vi "add pre post build to project.vi"(8 "error in (no error)":errorcluster, 11 "Builder":refnum<class "Builder.lvclass">) -> (0 "error out":errorcluster, 3 "Builder out":refnum<class "Builder.lvclass">)   [LabVIEW 2024, in "Builder.lvclass"]
doc: "If the path is valid, adds the pre and post build spec action vis to the open lv project"
uses:
  builders/parent/Builder.lvclass
  builders/parent/Builder.lvclass/Builder.ctl
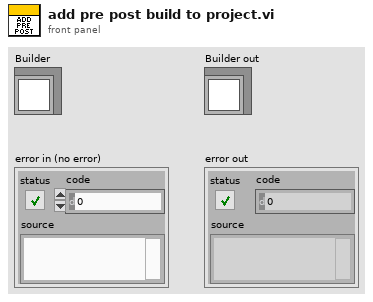
[diagram p1: front panel]
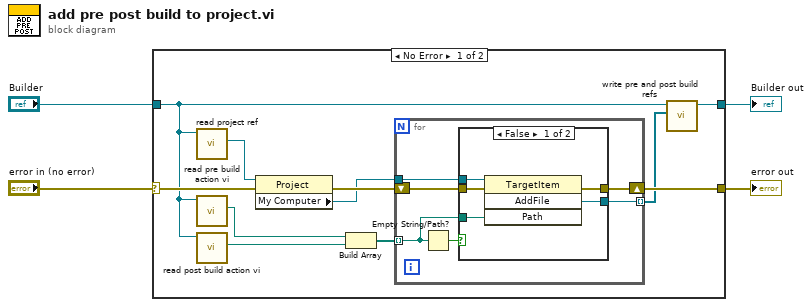
[diagram p0: block diagram]
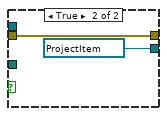
[diagram p2: hidden frame]
diagram:
  n1 = case shown="No Error" "error in (no error)" {
    selector: "error in (no error)" -> [w14 w30]
    tunnel: [w15 w30] -> w4
    tunnel: "Builder" -> [w6 w29]
    tunnel: [w8 w29] -> w1
    frame No Error {
      n2 = call "read project ref.vi"("Builders in"=w6) -> ("project ref"=w10:refnum<vi>)  [unwired: 10 in]
      n3 = call "read pre build action vi.vi"("Builder in"=w6) -> ("pre build action vi"=w7:path)  [unwired: 10 in]
      n4 = call "read post build action vi.vi"("Builder in"=w6) -> ("post build action vi"=w5:path)  [unwired: 10 in]
      n5 = property class="Project"(reference=w10, error in=w14) -> (error out=w12:errorcluster, "My Computer"=w11:refnum<vi>)  [unwired: 1 out]
      n6 = Build Array(w7, w5) -> (w13:path[])
      n7 = for {
        tunnel: w11 -> [w21]
        tunnel: w13 -> [w18] mode=indexing
        tunnel: [w19] -> w9 mode=indexing
        shift-right: [w16] -> w15
        shift-left: w12 -> [w20]
        n8 = Empty String/Path?(string/path=w18) -> (empty?=w17:bool)
        n9 = case shown="False" w17 {
          tunnel: w21 -> [w26 _]
          tunnel: w20 -> [w25 w27]
          tunnel: w18 -> [w24 _]
          tunnel: [w23 refnum<vi> refnum ("AddFile")] -> w19
          tunnel: [w22 w27] -> w16
          frame False {
            n10 = invoke class="TargetItem" method="AddFile"(reference=w26, error in=w25, "Path"=w24) -> (error out=w22:errorcluster, "AddFile"=w23:refnum<vi>)  [unwired: 1 in, 2 out]
          }
          frame True {
          }
        }
      }
      n11 = call "write pre and post build refs .vi"("pre and post build refs"=w9, "Builders in"=w6) -> ("Builders out"=w8:refnum<class "Builder.lvclass">)  [unwired: 9 in]
    }
    frame Error {
    }
  }
  "error out" <- w4
  "Builder out" <- w1
